vi "state告警数据存储.vi"(8 "错误输入（无错误）":errorcluster, 10 "data":T1, 11 "state":string) -> (0 "错误输出":errorcluster)   [LabVIEW 2022 SP3, in "Alarm interface.lvlib"]
uses:
  Alarm interface.lvlib
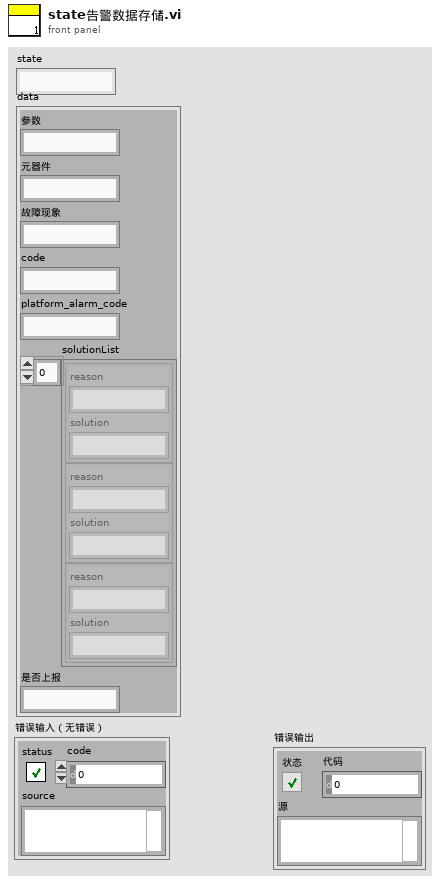
[diagram p1: front panel]
types:
  T1 = typedef "Alarm interface.lvlib/报警短信语音交互.ctl" = cluster{"参数":string, "元器件":string, "故障现象":string, "code":string, "platform_alarm_code":string, "solutionList":cluster{"reason":string, "solution":string}[], "是否上报":string}
  T2 = typedef "报警信息字段定义.ctl" = cluster{"时间":timestamp, "参数":string, "元器件":string, "故障现象":string, "故障分析":string, "state":string, "code":string, "platform_alarm_code":string, "是否上报":string}
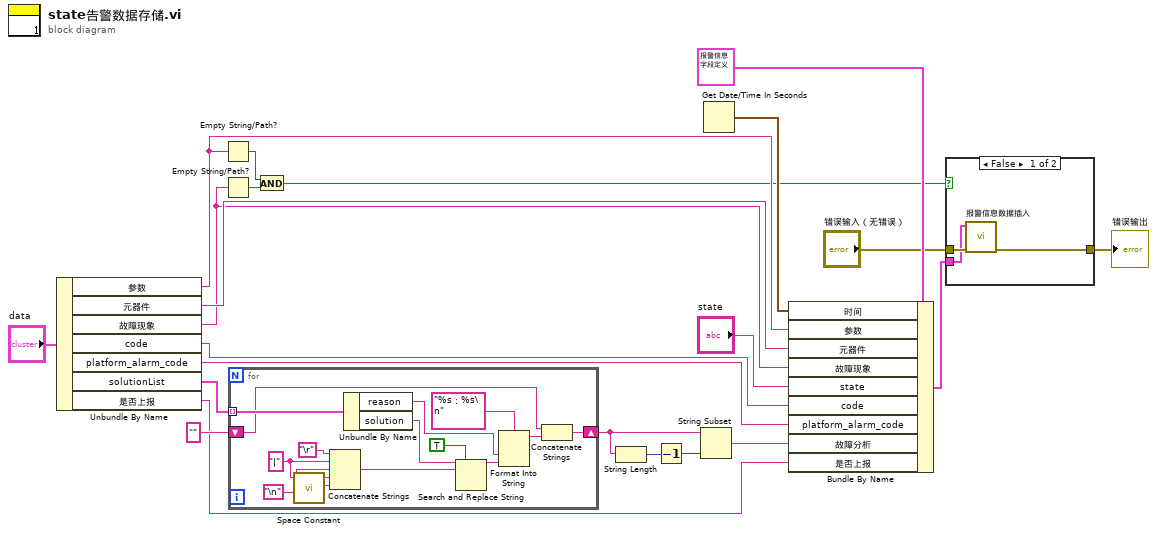
[diagram p0: block diagram]
diagram:
  n1 = Unbundle By Name("data") -> ("参数"=w7:string, "元器件"=w11:string, "故障现象"=w6:string, "code"=w12:string, "platform_alarm_code"=w13:string, "solutionList"=w15:cluster{"reason":string, "solution":string}[], "是否上报"=w1:string)
  n2 = Empty String/Path?(string/path=w7) -> (empty?=w5:bool)
  n3 = Empty String/Path?(string/path=w6) -> (empty?=w4:bool)
  n4 = for {
    tunnel: w15 -> [w36] mode=indexing
    shift-right: [w31] -> w16
    shift-left: "" -> [w32]
    w24 = "|" ("字符串")
    n5 = call <vilib>:"Space Constant.vi"() -> ("String"=w23:string)
    n6 = Concatenate Strings("\r", w24, "\n", w24, w23) -> (w27:string)
    n7 = Unbundle By Name(w36) -> ("reason"=w34:string, "solution"=w30:string)
    n8 = Search and Replace String(replace all?=TRUE ("替换全部？(F)"), input string=w30, search string=w27) -> (result string=w25:string)  [unwired: 5 in, 3 out]
    n9 = Format Into String(format string="%s：%s\n" ("格式字符串"), w34, w25) -> (resulting string=w33:string)  [unwired: 2 in, 1 out]
    n10 = Concatenate Strings(w32, w33) -> (w31:string)
  }
  n11 = And(x=w5, y=w4) -> (x .and. y?=w3:bool)
  n12 = String Length(string=w16) -> (length=w17:i32)
  n13 = Decrement(x=w17) -> (x-1=w18:i32)
  n14 = String Subset(string=w16, length (rest)=w18) -> (substring=w19:string)  [unwired: 1 in]
  n15 = Get Date/Time In Seconds() -> (seconds since 1Jan1904=w10:timestamp)
  n16 = Bundle By Name(cluster=T2 {"时间"=timestamp(0 s since 1904-01-01), "参数"="", "元器件"="", "故障现象"="", "故障分析"="", "state"="", "code"="", "platform_alarm_code"="", "是否上报"=""} ("data"), "时间"=w10, "参数"=w7, "元器件"=w11, "故障现象"=w6, "state"="state", "code"=w12, "platform_alarm_code"=w13, "故障分析"=w19, "是否上报"=w1) -> (w2:T2)
  n17 = case shown="False" w3 {
    tunnel: [w37 w40] -> w22
    tunnel: "错误输入（无错误）" -> [w39 w40]
    tunnel: w2 -> [w38 _]
    frame False {
      n18 = call "报警信息数据插入.vi"("data"=w38, "错误输入（无错误）"=w39) -> ("错误输出"=w37:errorcluster)  [unwired: 8 in]
    }
    frame True {
    }
  }
  "错误输出" <- w22
